vi "error_out.vi"(8 "error in (no error)":cluster{"状态":bool, "代码":i32, "源":string} caption="错误输入（无错误）", 9 "message":string="密码错误！", 10 "link":string="密码错误！", 11 "LabVIEW Web服务请求":refnum<class "Web Request.lvclass">) -> (0 "error out":cluster{"状态":bool, "代码":i32, "源":string} caption="错误输出", 3 "LabVIEW Web服务请求输出":refnum<class "Web Request.lvclass">)   [LabVIEW 2017]
uses:
  <vilib>/wsapi/Web Request.lvclass
  <vilib>/wsapi/class/subVIs/Set String ESP Variable.vi
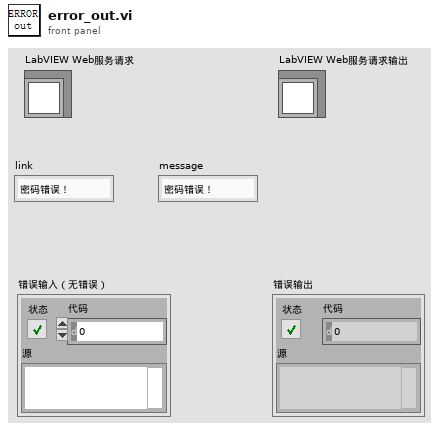
[diagram p1: front panel]
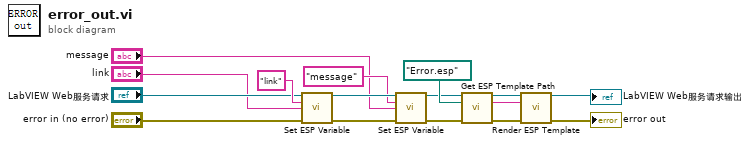
[diagram p0: block diagram]
diagram:
  n1 = call-poly <vilib>:"Set ESP Variable.vi"("LabVIEW Web Service Request"="LabVIEW Web服务请求", "key"="link", "value"="link", "error in (no error)"="error in (no error)") -> ("LabVIEW Web Service Request out"=w12:refnum<class "Web Request.lvclass">, "error out"=w9:errorcluster)  [unwired: 10 in]
  n2 = call-poly <vilib>:"Set ESP Variable.vi"("LabVIEW Web Service Request"=w12, "key"="message", "value"="message", "error in (no error)"=w9) -> ("LabVIEW Web Service Request out"=w7:refnum<class "Web Request.lvclass">, "error out"=w8:errorcluster)  [unwired: 10 in]
  n3 = call "Get ESP Template Path.vi"("LabVIEW Web服务请求"=w7, "模板相对路径"=path "Error.esp", "error in (no error)"=w8) -> ("LabVIEW Web服务请求输出"=w16:refnum<class "Web Request.lvclass">, "模板名称"=w15:string, "error out"=w14:cluster{"状态":bool, "代码":i32, "源":string})  [unwired: 10 in]
  n4 = call <vilib>:"Render ESP Template.vi"("LabVIEW Web Service Request"=w16, "espName"=w15, "error in (no error)"=w14) -> ("LabVIEW Web Service Request out"=→"LabVIEW Web服务请求输出":refnum<class "Web Request.lvclass">, "error out"=→"error out":errorcluster)  [unwired: 11 in]
